vi "JsonFile_SetAttribute(String).vi"(8 "error in (no error)":errorcluster, 9 "Value":string, 10 "Attribute":string, 11 "Json":path) -> (0 "error out":errorcluster, 3 "Json (dup)":path)   [LabVIEW 2019, in "lv-apt-json-file.lvlib"]
uses:
  <userlib>/_lvAPT/lv-apt-json-file/lv-apt-json-file.lvlib
  <vilib>/addons/_JKI.lib/Serialization/JSON/JKI JSON Serialization.lvlib
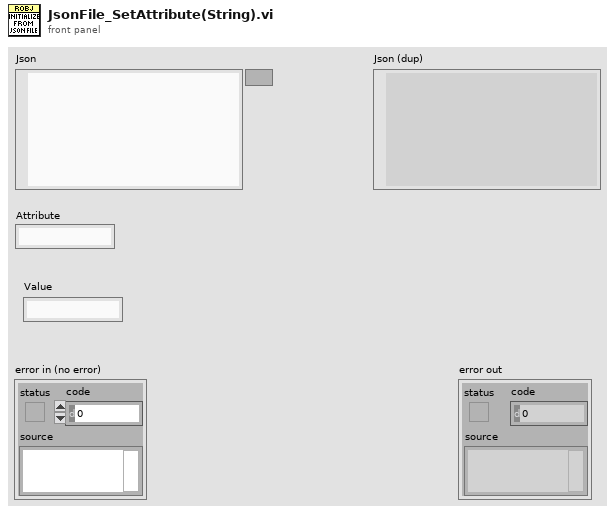
[diagram p1: front panel]
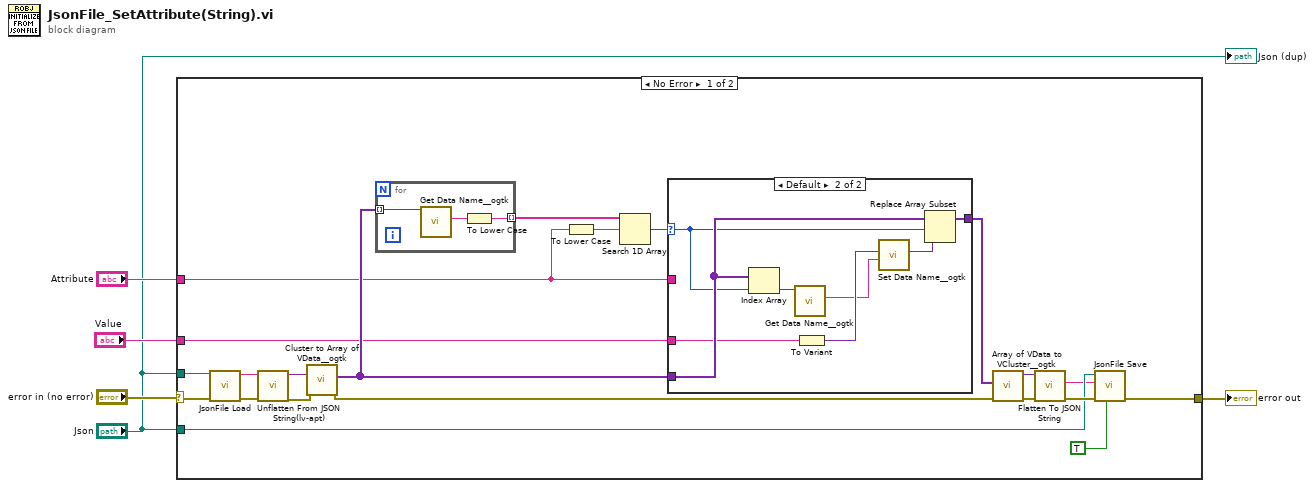
[diagram p0: block diagram]
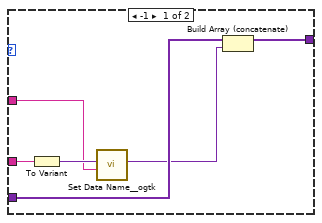
[diagram p2: hidden frame]
diagram:
  n1 = case shown="No Error" "error in (no error)" {
    selector: "error in (no error)" -> [w22 w44]
    tunnel: "Json" -> [w21 _]
    tunnel: [w19 w44] -> w4
    tunnel: "Attribute" -> [w6 _]
    tunnel: "Value" -> [w16 _]
    tunnel: "Json" -> [w9 _]
    frame No Error {
      n2 = call <userlib>:"JsonFile Load.vi"("error in (no error)"=w22, "Path"=w21) -> ("error out"=w24:errorcluster, "Json"=w23:string)  [unwired: 8 in]
      n3 = call <userlib>:"Unflatten From JSON String(lv-apt).vi"("error in (no error)"=w24, "JSON String"=w23) -> ("error out"=w26:errorcluster, "Variant"=w25:variant)  [unwired: 8 in]
      n4 = call <userlib>:"Cluster to Array of VData__ogtk.vi"("error in (no error)"=w26, "Cluster"=w25) -> ("error out"=w20:errorcluster, "Array of VData"=w17:variant[])  [unwired: 8 in]
      n5 = for {
        tunnel: w17 -> [w43] mode=indexing
        tunnel: [w42] -> w18 mode=indexing
        n6 = call <userlib>:"Get Data Name__ogtk.vi"("Data"=w43) -> ("Data Name"=w41:string)  [unwired: 8 in, 2 out]
        n7 = To Lower Case(string=w41) -> (all lower case string=w42:string)
      }
      n8 = To Lower Case(string=w6) -> (all lower case string=w15:string)
      n9 = Search 1D Array(1D array=w18, element=w15) -> (index of element=w14:i32)  [unwired: 1 in]
      n10 = case shown="Default" w14 {
        selector: w14 -> [_ w38]
        tunnel: w17 -> [w29 w40]
        tunnel: w16 -> [w32 w39]
        tunnel: [w28 w33] -> w13
        tunnel: w6 -> [w30 _]
        frame -1 {
          n11 = To Variant(anything=w32) -> (Variant=w31:variant)
          n12 = call <userlib>:"Set Data Name__ogtk.vi"("Data Name"=w30, "Data"=w31) -> ("Renamed Data"=w27:variant)  [unwired: 8 in, 1 out]
          n13 = Build Array (concatenate)(w29, w27) -> (w28:variant[])
        }
        frame Default {
          n14 = Index Array(array=w40, index=w38) -> (element=w35:variant)
          n15 = call <userlib>:"Get Data Name__ogtk.vi"("Data"=w35) -> ("Data Name"=w34:string)  [unwired: 8 in, 2 out]
          n16 = To Variant(anything=w39) -> (Variant=w37:variant)
          n17 = call <userlib>:"Set Data Name__ogtk.vi"("Data Name"=w34, "Data"=w37) -> ("Renamed Data"=w36:variant)  [unwired: 8 in, 1 out]
          n18 = Replace Array Subset(array=w40, new element=w36, index=w38) -> (w33:variant[])
        }
      }
      n19 = call <userlib>:"Array of VData to VCluster__ogtk.vi"("error in (no error)"=w20, "Array"=w13) -> ("error out"=w12:errorcluster, "VCluster"=w10:variant)  [unwired: 8 in]
      n20 = call <vilib>:"Flatten To JSON String.vi"("error in (no error)"=w12, "Variant"=w10) -> ("error out"=w11:errorcluster, "JSON String"=w8:string)  [unwired: 8 in]
      n21 = call <userlib>:"JsonFile Save.vi"("Pretty Print(T)"=TRUE, "error in (no error)"=w11, "JSON String"=w8, "Path"=w9) -> ("error out"=w19:errorcluster)  [unwired: 7 in]
    }
    frame Error {
    }
  }
  "error out" <- w4
  "Json (dup)" <- "Json"
